vi "Start API.vi"(7 "Shutter":T1={"Open command string"="+100\\s10\\n", "VISA"={"Timeout (ms)"=10000, "Resource Name"="COM1", "Baud Rate"=9600, "Data Bits"=8, "Parity"=0, "Stop Bits"=10, "Flow Control"=0}} {"VISA"."Flow Control" items=["None"=0, "XON/XOFF"=1, "RTS/CTS"=2, "DTR/DSR"=4]; "VISA"."Stop Bits" items=["1.0"=10, "1.5"=15, "2.0"=20]; "VISA"."Parity" items=["None", "Odd", "Even", "Mark", "Space"]}, 8 "Error In":errorcluster) -> (0 "Error Out":errorcluster)   [LabVIEW 2017, in "Shutter.lvlib"]
uses:
  Shutter.lvlib
  Controls/Params.ctl
  Monochromator/Controls/VISA parameters.ctl
  Controls/Module Command Data [cluster].ctl
  Controls/Module Commands [enum].ctl
  Events/Events.lvlib
  Serial comms/Serial comms.lvlib
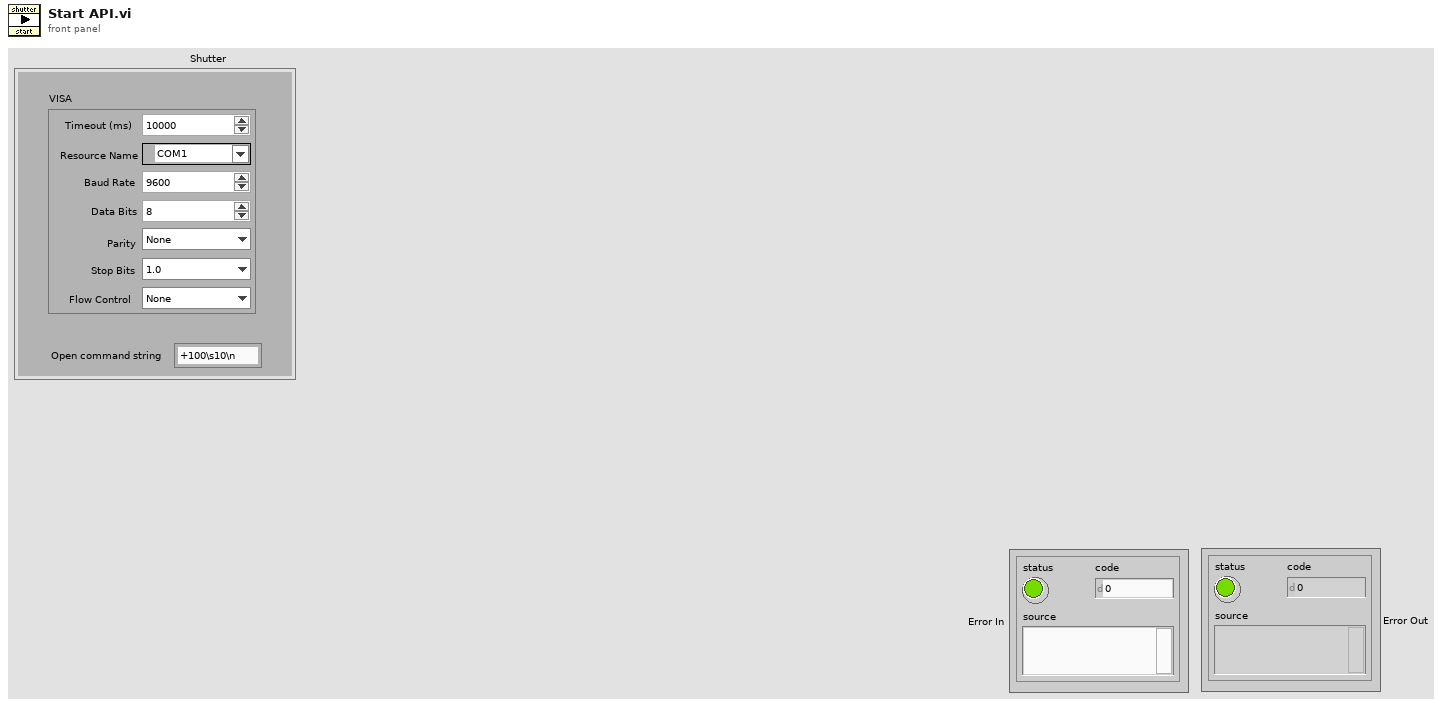
[diagram p1: front panel]
types:
  T1 = typedef "Shutter.lvlib/Params.ctl" = cluster{"Open command string":string, "VISA":T2}
  T2 = typedef "Serial comms.lvlib/VISA parameters.ctl" = cluster{"Timeout (ms)":u32, "Resource Name":refnum<visa-resource-name>, "Baud Rate":u32, "Data Bits":u16, "Parity":u16, "Stop Bits":u16, "Flow Control":u16}
  T3 = typedef "Shutter.lvlib/Module Command Data [cluster].ctl" = cluster{"Command":T4, "Data":variant}
  T4 = typedef "Shutter.lvlib/Module Commands [enum].ctl" = enum16{"Start", "Move", "Return", "Stop"}
  T5 = typedef "Events.lvlib/Refs [cluster].ctl" = cluster{"Exit":refnum<user-event>, "Controller":refnum<user-event>, "System Error":refnum<user-event>, "UI":refnum<user-event>, "Example Module":refnum<user-event>, "Shutter":refnum<user-event>, "Monochromator":refnum<user-event>, "DAQ":refnum<user-event>, "Scope":refnum<user-event>, "Processing":refnum<user-event>, "File IO":refnum<user-event>, "Colour wheel":refnum<user-event>}
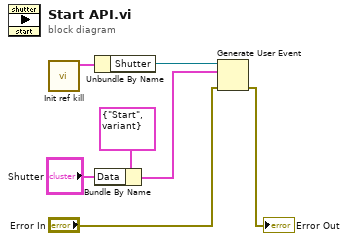
[diagram p0: block diagram]
diagram:
  n1 = call "Init ref kill.vi"() -> ("Messages"=w7:T5)  [unwired: 10 in, 1 out]
  n2 = Unbundle By Name(w7) -> ("Shutter"=w6:refnum<user-event>)
  n3 = Bundle By Name(cluster=T3 {"Command"=enum."Start", "Data"=variant} ("event data"), "Data"="Shutter") -> (w3:T3)
  n4 = Generate User Event(user event=w6, event data cluster=w3, error in="Error In") -> (error out=→"Error Out":errorcluster)  [unwired: 1 in, 1 out]
